vi "B-Spline Fit.vi"   [LabVIEW 2024, in "NI_AALPro.lvlib"]
doc: "<p>Uses B-spline fitting to smooth a data set.</p>"
uses:
  NI_AALPro.lvlib
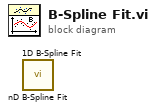
[diagram p0: block diagram]
diagram:
  n1 = call "nD B-Spline Fit.vi"() -> ()  [unwired: 13 in, 3 out]
  n2 = call "1D B-Spline Fit.vi"() -> ()  [unwired: 12 in, 4 out]
